vi "JsonTemplate Main.vi"(11 "Tag IN":T1={"Tag Name"=["LStatus", "RStatus", "LTargetTemp", "LTemp1", "LTemp2", "LTemp3", "LTemp4", "LTemp5", "LTemp6", "RTargetT", "RTemp1", "RTemp2", "RTemp3", "RTemp4", "RTemp5", "RTemp6", "LWO", "LOPID", "LDate", "LTime", "LModel", "LAgingTime", "LAgingTemp", "LStartTime", "LEndTime", "RWO", "ROPID", "RDate", "RTime", "RModel", "RAgingTime", "RAgingTemp", "RStartTime", "REndTime"], "Tag Type"=[enum."String", enum."String", enum."Double", enum."Double", enum."Double", enum."Double", enum."Double", enum."Double", enum."Double", enum."Double", enum."Double", enum."Double", enum."Double", enum."Double", enum."Double", enum."Double", enum."String", enum."String", enum."String", enum."String", enum."String", enum."String", enum."String", enum."String", enum."String", enum."String", enum."String", enum."String", enum."String", enum."String", enum."String", enum."String", enum."String", enum."String"], "Tag Data"=[], "Skyline Array"=[]}) -> (3 "output cluster":T1={"Tag Name"=["LStatus", "RStatus", "LTargetTemp", "LTemp1", "LTemp2", "LTemp3", "LTemp4", "LTemp5", "LTemp6", "RTargetT", "RTemp1", "RTemp2", "RTemp3", "RTemp4", "RTemp5", "RTemp6", "LWO", "LOPID", "LDate", "LTime", "LModel", "LAgingTime", "LAgingTemp", "LStartTime", "LEndTime", "RWO", "ROPID", "RDate", "RTime", "RModel", "RAgingTime", "RAgingTemp", "RStartTime", "REndTime"], "Tag Type"=[enum."String", enum."String", enum."Double", enum."Double", enum."Double", enum."Double", enum."Double", enum."Double", enum."Double", enum."Double", enum."Double", enum."Double", enum."Double", enum."Double", enum."Double", enum."Double", enum."String", enum."String", enum."String", enum."String", enum."String", enum."String", enum."String", enum."String", enum."String", enum."String", enum."String", enum."String", enum."String", enum."String", enum."String", enum."String", enum."String", enum."String"], "Tag Data"=[], "Skyline Array"=[]})   [LabVIEW 2017]
uses:
  Tag.ctl
  <vilib>/Skyline/Tag/Shared/typedefs/DataType.ctl
  <vilib>/Skyline/Tag/Wrapper/Wrapper_class/NI Skyline Tag.lvclass
  <vilib>/Skyline/Tag/Shared/NI Skyline Tag.lvlib
panel:
  in  "initialized array 2":variant[](array[variant])
  in  "initialized array":variant[](array[variant])
  out "Numeric Control":i32
  out "Array 2":string[](array[string])
  out "Array":variant[](array[variant])
  in  "Cluster":T3={"ChamberStatus"={"LStatus"="Idle", "RStatus"="Idle"}, "Temperature"={"LTargetTemp"=0.0, "LTemp"=[26.2, 26.6, 25.9, 24.9, 25.5, 25.6], "RTargetTemp"=0.0, "RTemp"=[26.3, 26.3, 26.3, 26.3, 28.0, 27.5]}, "Operation Status"={"LOperationStatus"=",,2018-07-03,17:08:55,[100]_(0)(45)-100,0,0,,", "ROperationStatus"=",,2018-07-03,17:08:55,[100]_(0)(45)-100,0,0,0,0"}, "BIB Board Number"={"LBoardNumber"=",,,,,,,,,,,,,,,,,,,,,,,,,", "RBoardNumber"=",,,,,,,,,,,,,,,,,,,,,,,,,"}, "Connect Position Information"="0683=0,0,0,129,0,129,0,0,0,0,0,0,0,0,0,0,0,0,129,255,0,255,0,0,0,0,0,0,0,0,0,0\n0544=0,0,0,0,255,0,0,0,0,0,0,0,0,0,0,0,0,0,0,0,0,0,0,0,0,0,0,147,0,0,0,0\n0548=0,0,0,0,0,18,0,0,0,255,0,0,0,0,0,147,0,0,0,255,0,255,81,255,255,255,255,255,255,255,255,0\n0690=0,0,0,0,255,255,255,255,0,0,0,0,0,0,0,0,0,129,0,0,147,0,0,0,0,0,146,0,0,0,0,0\n0688=0,0,0,147,0,0,0,0,0,147,129,0,0,0,0,0,129,0,0,0,0,0,147,0,147,0,0,129,0,0,0,0\n0684=129,0,0,0,0,0,0,0,0,0,0,0,255,0,0,0,0,0,147,0,0,0,0,0,0,0,0,0,0,0,0,255\n0692=129,0,0,0,0,0,0,0,0,0,0,255,0,0,0,0,0,0,0,0,0,0,0,0,255,0,0,0,129,0,0,0\n0116=0,0,0,0,0,0,0,255,0,0,0,0,0,0,0,0,0,0,0,129,129,0,17,0,0,129,0,0,0,0,0,0\n0523=0,0,0,0,0,0,0,0,0,0,0,0,0,0,0,0,0,0,0,0,255,255,255,255,255,255,255,255,255,255,255,255\n"}
  out "Connect Position Information":dbl[][](array[numeric])
  out "RBoardNumber":string[](array[string])
  out "LBoardNumber":string[](array[string])
  out "JSON string":string
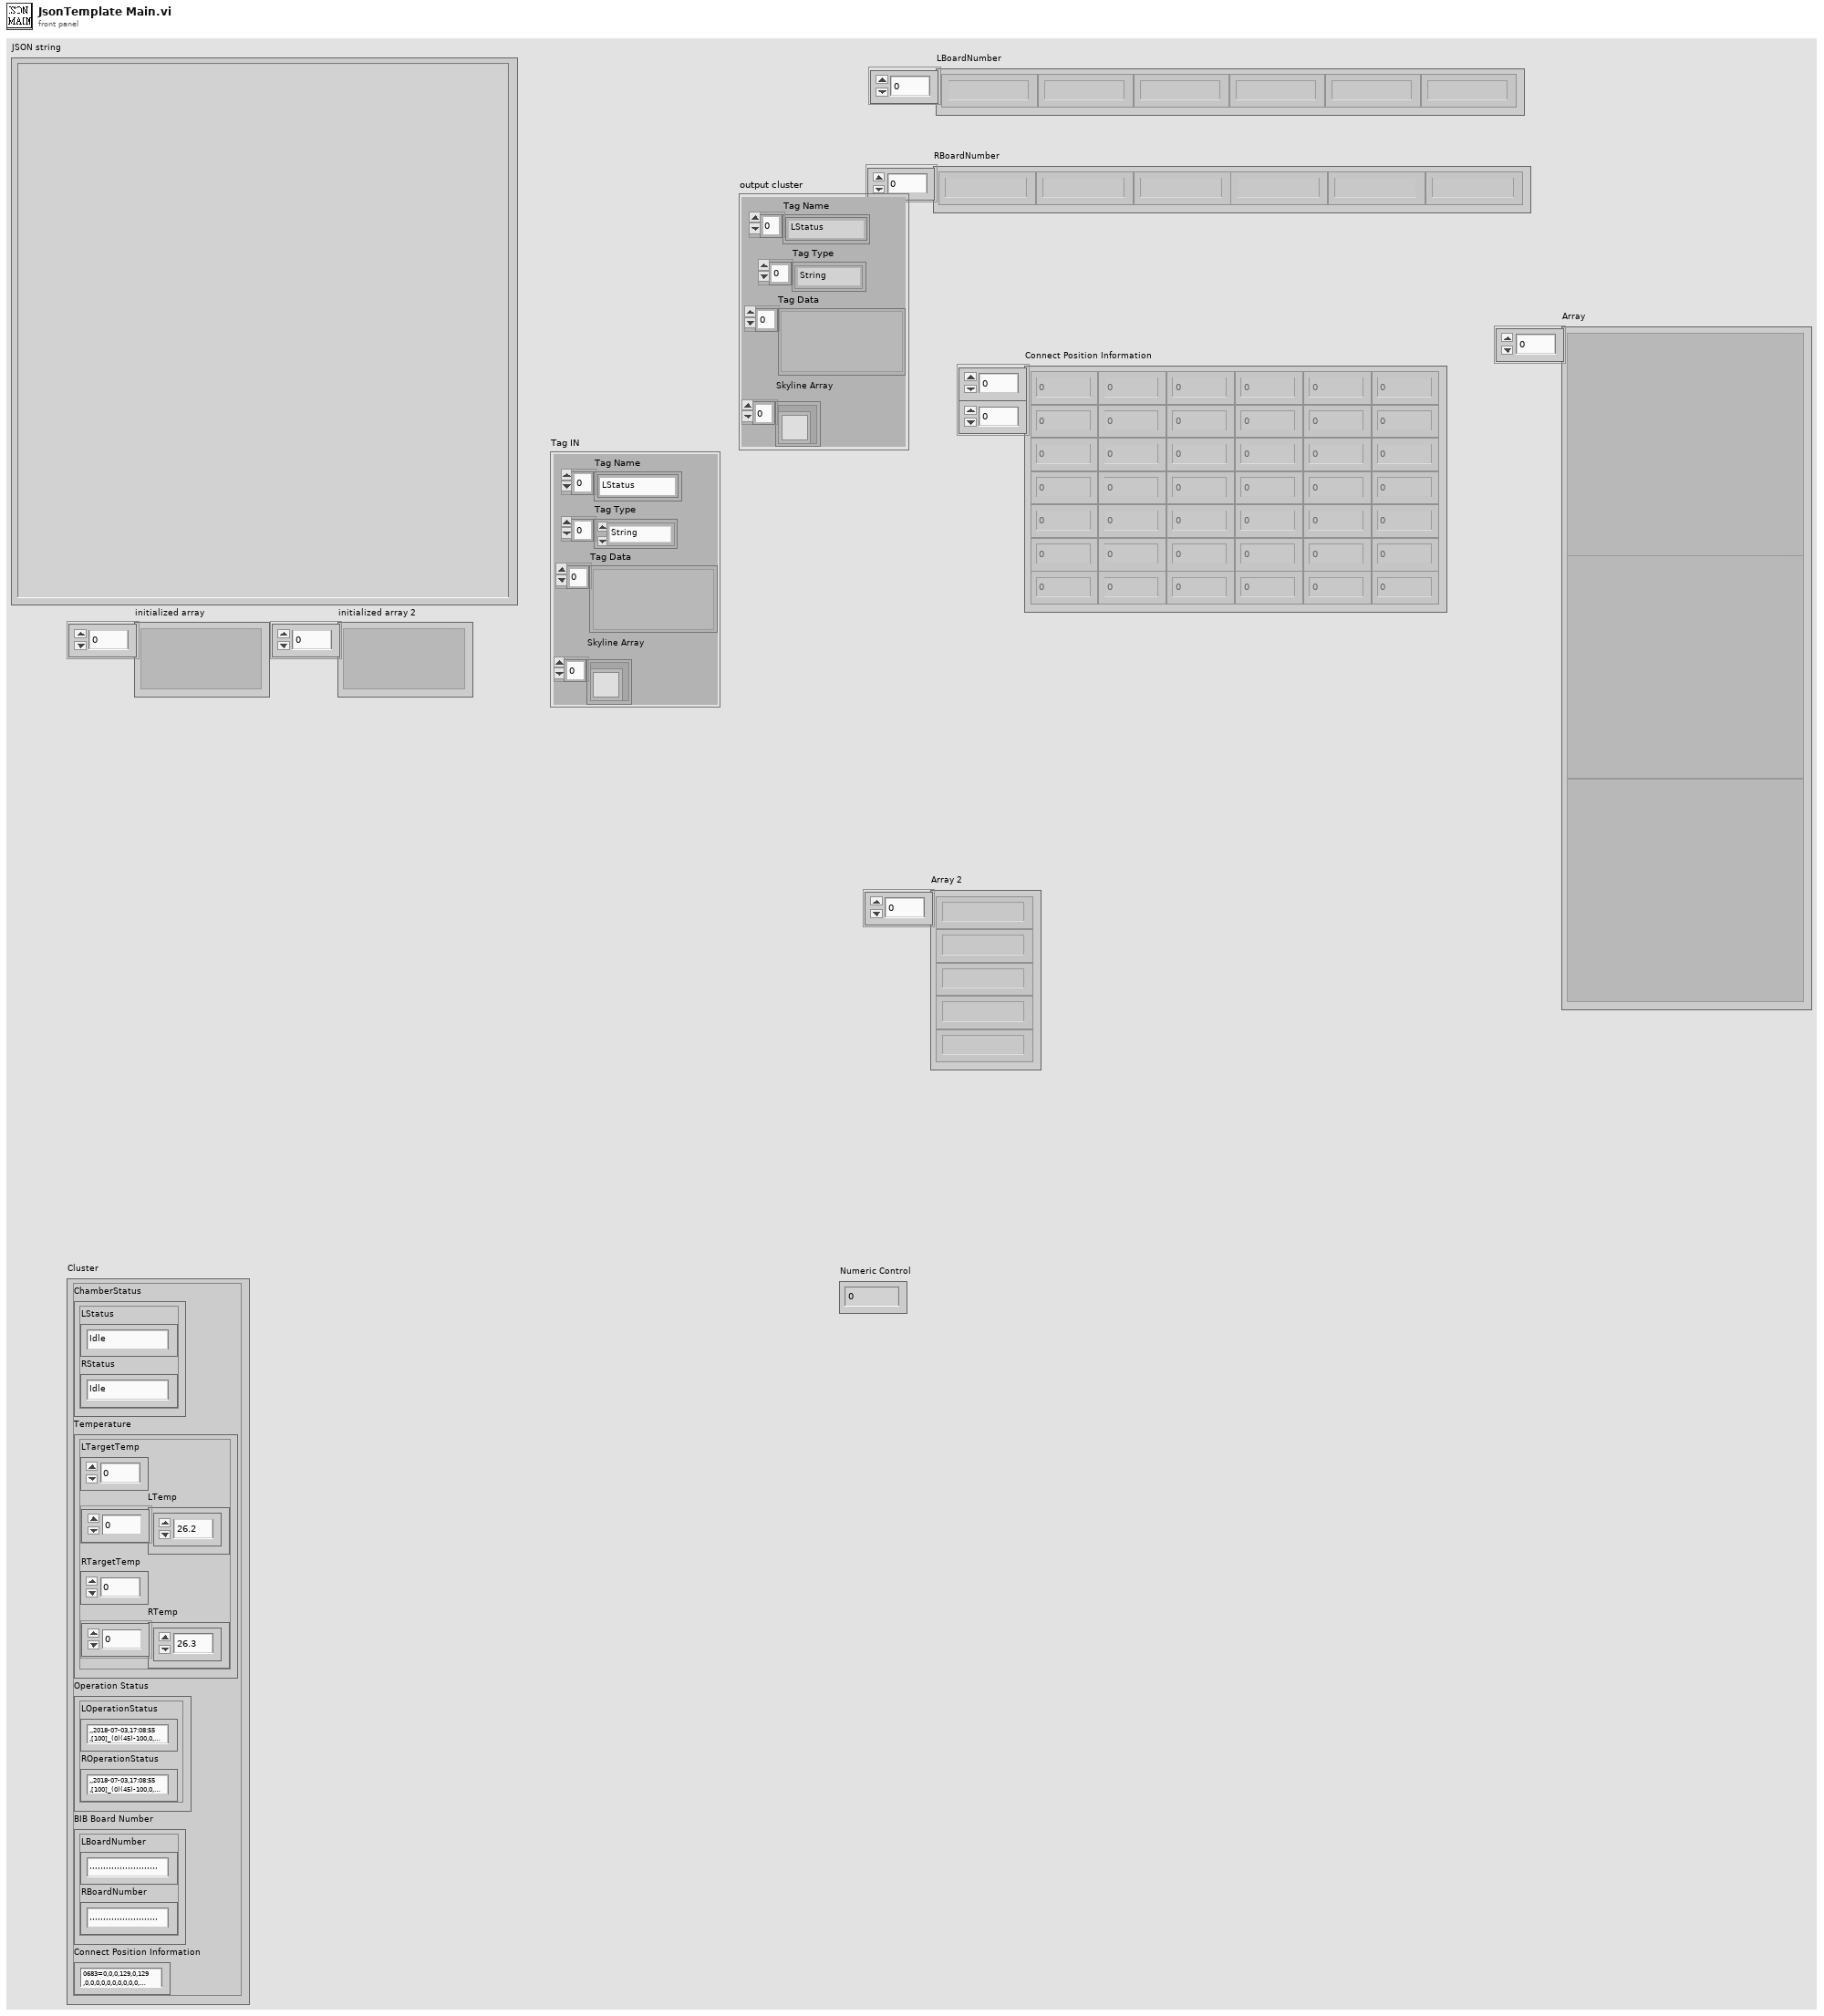
[diagram p1: front panel]
types:
  T1 = typedef "Tag.ctl" = cluster{"Tag Name":string[], "Tag Type":T2[], "Tag Data":variant[], "Skyline Array":refnum<class "NI Skyline Tag.lvclass">[]}
  T2 = typedef "NI Skyline Tag.lvlib/DataType.ctl" = enum32{"Double", "I32", "String", "Boolean", "U64", "Timestamp"}
  T3 = cluster{"ChamberStatus":cluster{"LStatus":string, "RStatus":string}, "Temperature":cluster{"LTargetTemp":dbl, "LTemp":dbl[], "RTargetTemp":dbl, "RTemp":dbl[]}, "Operation Status":cluster{"LOperationStatus":string, "ROperationStatus":string}, "BIB Board Number":cluster{"LBoardNumber":string, "RBoardNumber":string}, "Connect Position Information":string}
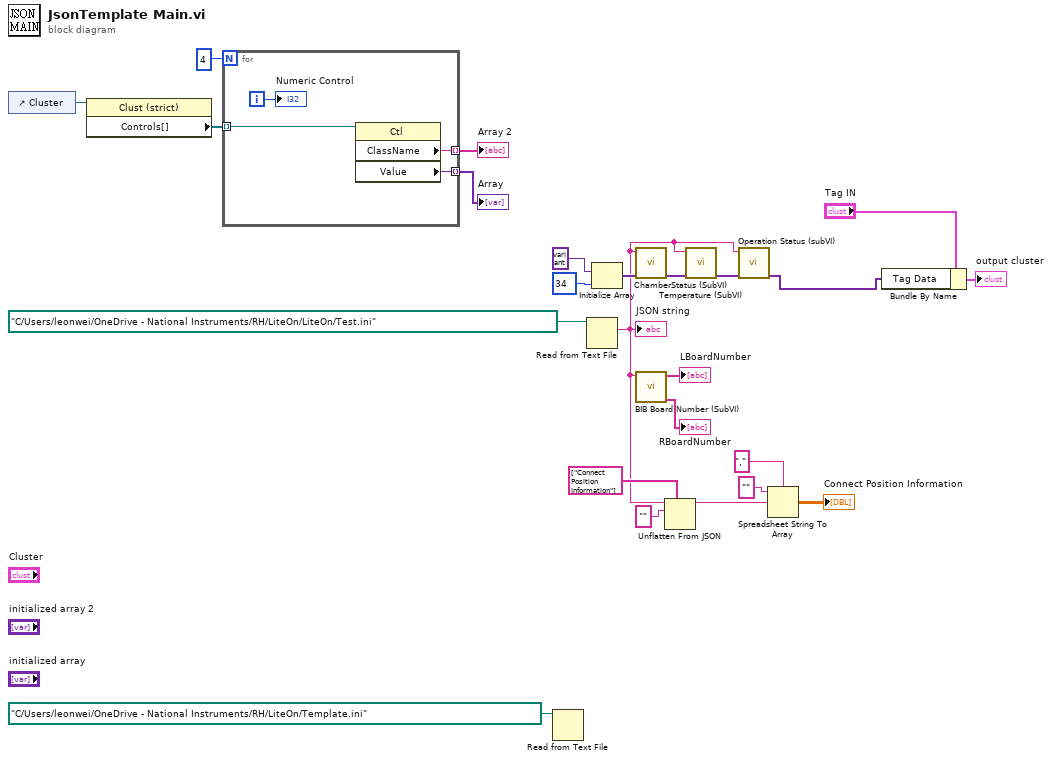
[diagram p0: block diagram]
diagram:
  n1 = control-ref of="Cluster"() -> (w15:refnum<vi>)
  n2 = property on="Property Node" class="Clust (strict)"(reference=w15) -> ("Controls[]"=w16:refnum<vi>[])  [unwired: 1 in, 2 out]
  n3 = for {
    N: 4 -> [_]
    tunnel: w16 -> [w28] mode=indexing
    tunnel: [w27] -> w14 mode=indexing
    tunnel: [w25] -> w11 mode=indexing
    i -> [w26]
    n4 = property class="Ctl"(reference=w28) -> ("ClassName"=w27:string, "Value"=w25:variant)  [unwired: 1 in, 2 out]
    "Numeric Control" <- w26
  }
  "Array" <- w11
  "Array 2" <- w14
  n5 = Read from Text File(file (use dialog)=path "C:/Users/leonwei/OneDrive - National Instruments/RH/LiteOn/Template.ini") -> ()  [unwired: 3 in, 4 out]
  n6 = Read from Text File(file (use dialog)=path "C:/Users/leonwei/OneDrive - National Instruments/RH/LiteOn/LiteOn/Test.ini") -> (text=w4:string)  [unwired: 3 in, 3 out]
  "JSON string" <- w4
  n7 = Initialize Array(variant, 34 ("dimension size")) -> (w8:variant[])
  n8 = call "ChamberStatus (SubVI).vi"("initialized array"=w8, "JSON string"=w4) -> ("output array"=w7:variant[])  [unwired: 9 in]
  n9 = call "BIB Board Number (SubVI).vi"("JSON string"=w4) -> ("ROperationStatus"=→"RBoardNumber":string[], "LOperationStatus"=→"LBoardNumber":string[])  [unwired: 9 in]
  n10 = Unflatten From JSON(path=string[] ["Connect Position Information"], JSON string=w4, type and defaults="") -> (value=w20:string)  [unwired: 4 in, 1 out]
  n11 = call "Temperature (SubVI).vi"("Input Array"=w7, "JSON string"=w4) -> ("output array"=w6:variant[])  [unwired: 9 in]
  n12 = call "Operation Status (subVI).vi"("Input Array"=w6, "JSON string"=w4) -> ("output array"=w2:variant[])  [unwired: 9 in]
  n13 = Spreadsheet String To Array(delimiter (Tab)=",", format string="", spreadsheet string=w20) -> (array=→"Connect Position Information":dbl[][])  [unwired: 1 in]
  n14 = Bundle By Name(cluster="Tag IN", "Tag Data"=w2) -> (→"output cluster":T1)
